vi "Read chart cluster element.vi"(8 "error in (no error)":errorcluster, 9 "Chart cluster element":i32, 10 "Channel":i8=-1, 11 "Chart cluster":T3) -> (0 "error out":errorcluster, 1 "Chart ref":T1, 2 "Chart cluster":T2 {"ID" format="ch %d"}, 3 "Chart cluster":T3)   [LabVIEW 2016]
uses:
  Typedefs/Hit chart cluster refnum.ctl
  Typedefs/HitChart.ctl
  Typedefs/HitChart refnum.ctl
  Typedefs/single Hitchart cluster refnum.ctl
panel:
  # "You can specify the chart you want either by giving the index\nin the cluster (chart cluster element), or by specifying the channel\nwhich the chart corresponds to.\n\nIf you leave Chart cluster element blank, it will use Chart cluster element."
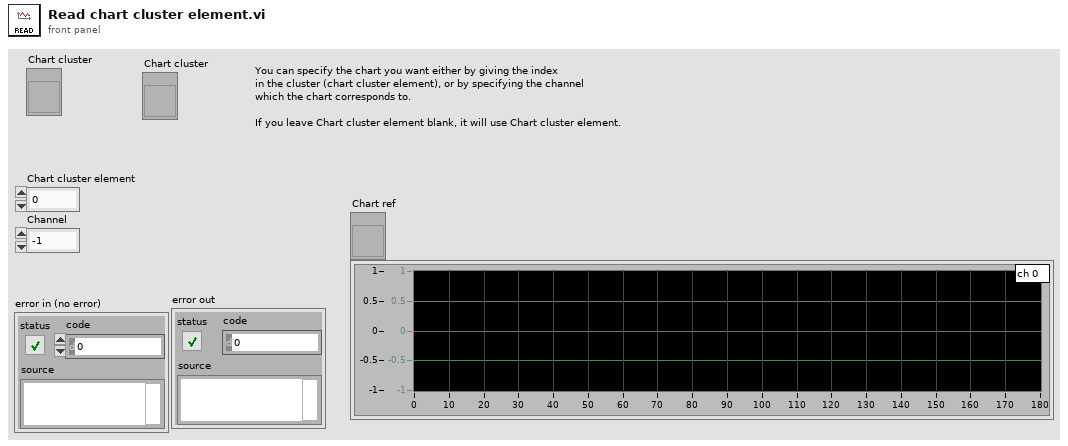
[diagram p1: front panel]
types:
  T1 = typedef "HitChart refnum.ctl" = refnum<vi>
  T2 = typedef "HitChart.ctl" = cluster{"Waveform Chart":cluster{"Coincidences":dbl, "Non-coincidences":dbl, "Ratio":dbl, "Total hits":dbl}[], "Last update timestamp":timestamp, "Resolution(s)":dbl, "nondisplayed coincs":i32, "nondisplayed noncoincs":i32, "Last upd":i64, "ID":i8}
  T3 = typedef "Hit chart cluster refnum.ctl" = refnum<vi>
  T4 = typedef "single Hitchart cluster refnum.ctl" = refnum<vi>
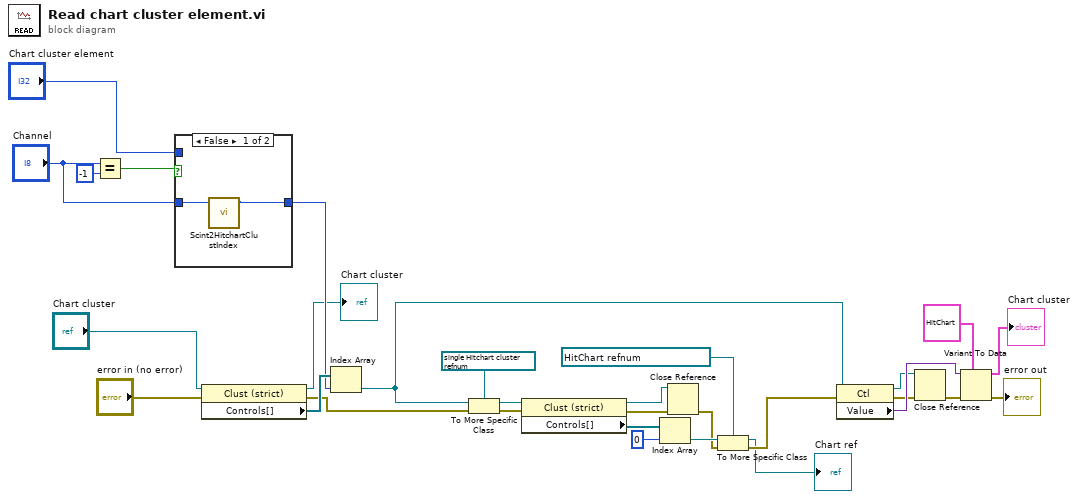
[diagram p0: block diagram]
diagram:
  n1 = Equal?(x="Channel", y=i8 -1) -> (x = y?=w12:bool)
  n2 = case shown="False" w12 {
    tunnel: "Channel" -> [w32 _]
    tunnel: [w31 w33] -> w28
    tunnel: "Chart cluster element" -> [_ w33]
    frame False {
      n3 = call "Scint2HitchartClustIndex.vi"("Channel"=w32) -> ("Numeric"=w31:i8)  [unwired: 10 in]
    }
    frame True {
    }
  }
  n4 = property class="Clust (strict)"(reference="Chart cluster", error in="error in (no error)") -> (reference out=→"Chart cluster":T3, error out=w15:errorcluster, "Controls[]"=w29:refnum<vi>[])
  n5 = Index Array(array=w29, index=w28) -> (element=w16:refnum<vi>)
  n6 = To More Specific Class(target class=T4 refnum ("Single hitchart"), reference=w16, error in=w15) -> (specific class reference=w10:T4, error out=w3:errorcluster)
  n7 = property class="Clust (strict)"(reference=w10, error in=w3) -> (reference out=w5:T4, error out=w6:errorcluster, "Controls[]"=w9:refnum<vi>[])
  n8 = Index Array(array=w9, index=0) -> (element=w7:refnum<vi>)
  n9 = Close Reference(reference=w5, error in (no error)=w6) -> (error out=w4:errorcluster)
  n10 = To More Specific Class(target class=T1 refnum ("Chart ref 2"), reference=w7, error in=w4) -> (specific class reference=→"Chart ref":T1, error out=w14:errorcluster)
  n11 = property class="Ctl"(reference=w16, error in=w14) -> (reference out=w22:refnum<vi>, error out=w23:errorcluster, "Value"=w27:variant)
  n12 = Close Reference(reference=w22, error in (no error)=w23) -> (error out=w21:errorcluster)
  n13 = Variant To Data(error in=w21, type=T2 {"Waveform Chart"=[], "Last update timestamp"=timestamp(0 s since 1904-01-01), "Resolution(s)"=0.0, "nondisplayed coincs"=0, "nondisplayed noncoincs"=0, "Last upd"=0, "ID"=0} ("Histogram cluster"), Variant=w27) -> (data=→"Chart cluster":T2, error out=→"error out":errorcluster)
